vi "comm write.vi"(8 "error in (no error)":errorcluster, 10 "string to write":string, 11 "Comm Handle":u64) -> (0 "error out":errorcluster, 2 "bytes written":u32, 3 "dup Comm Handle":u64)   [LabVIEW 2021, in "lvserial.lvlib"]
doc: "Writes data to the serial port."
uses:
  lvserial.lvlib
  lvserial.dll
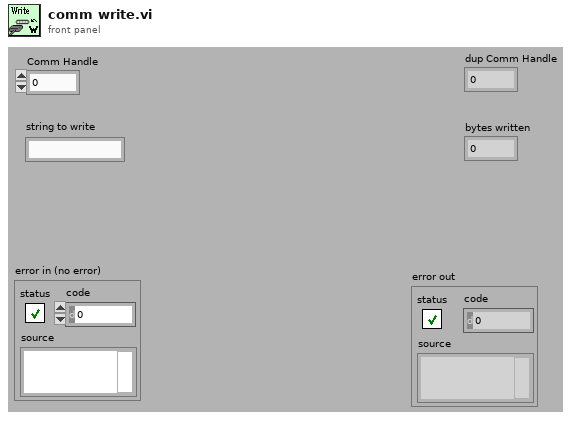
[diagram p1: front panel]
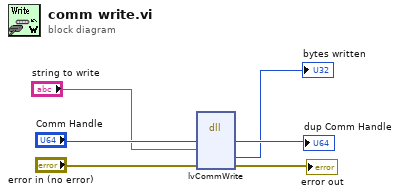
[diagram p0: block diagram]
diagram:
  n1 = dll-call lib="lvserial.dll" fn="lvCommWrite"("hComm"="Comm Handle", "Buffer"="string to write", "error"="error in (no error)") -> ("hComm"=→"dup Comm Handle":u64, "pulBytesWritten"=→"bytes written":u32, "error"=→"error out":errorcluster)  [unwired: 4 in, 4 out]
